vi "ProjectorCameraXY2LinearTransformation.vi"(7 "error in (no error)":errorcluster, 9 "ProjectorXY":cluster{"X":dbl, "Y":dbl}[](graph), 10 "CameraXY":cluster{"X":dbl, "Y":dbl}[](graph)) -> (0 "error out":errorcluster, 3 "Linear Tranformation Description":T1 {"mean error\n(projector pixels)" format="%0.2f"})   [LabVIEW 2019]
uses:
  LinearTransformationDescriptionCluster.ctl
  <vilib>/vision/NI_Vision_Development_Module.lvlib
panel:
  out "CameraXY 3":cluster{"X":dbl, "Y":dbl}[](graph)
  out "ProjectorXY 3":cluster{"X":sgl, "Y":sgl}[](graph)
  out "ProjectorXY 2":cluster{"X":dbl, "Y":dbl}[](graph)
  out "CameraToProjectorCorrectionFactor Y":dbl
  out "CameraToProjectorCorrectionFactor X":dbl
  out "Y axis error":sgl
  out "CameraXY 2":cluster{"X":dbl, "Y":dbl}[](graph)
  out "y axis relative to x":sgl
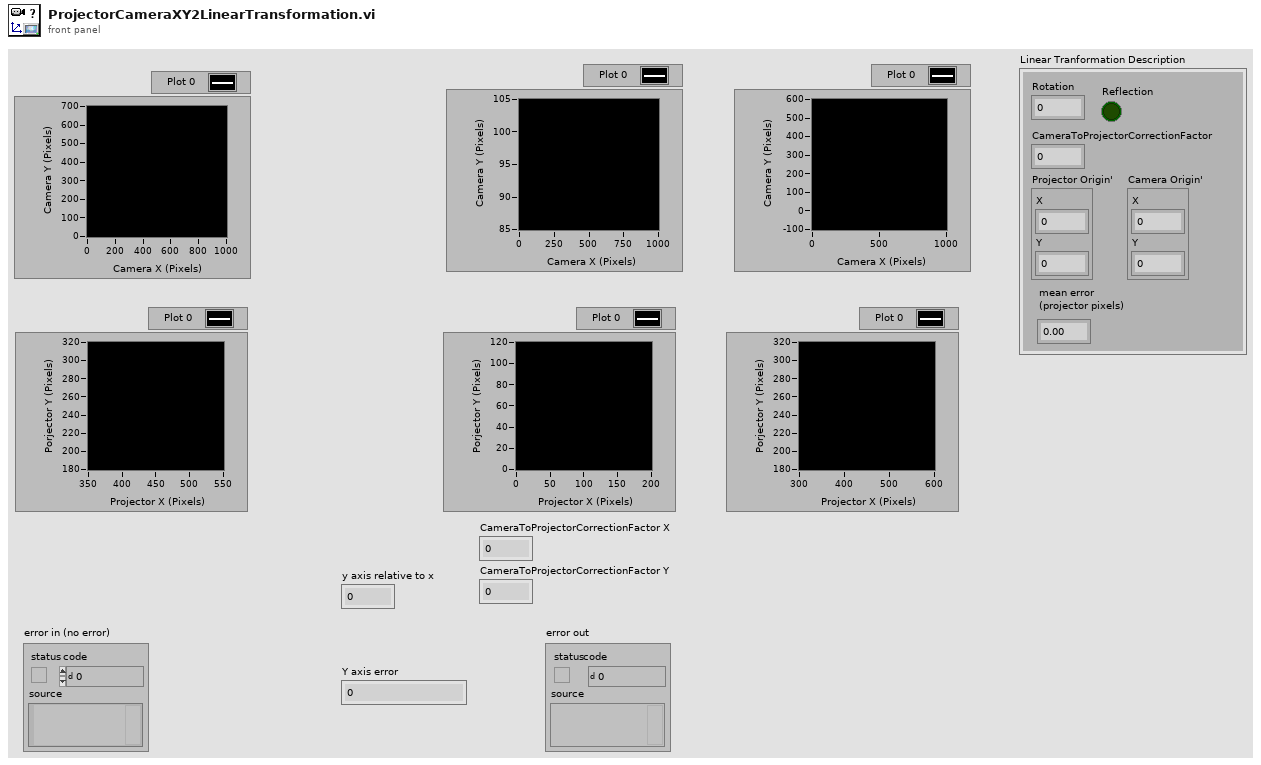
[diagram p1: front panel]
types:
  T1 = typedef "LinearTransformationDescriptionCluster.ctl" = cluster{"Rotation":sgl, "Reflection":bool, "CameraToProjectorCorrectionFactor":dbl, "Projector Origin'":cluster{"X":dbl, "Y":dbl}, "Camera Origin'":cluster{"X":dbl, "Y":dbl}, "mean error\n(projector pixels)":dbl}
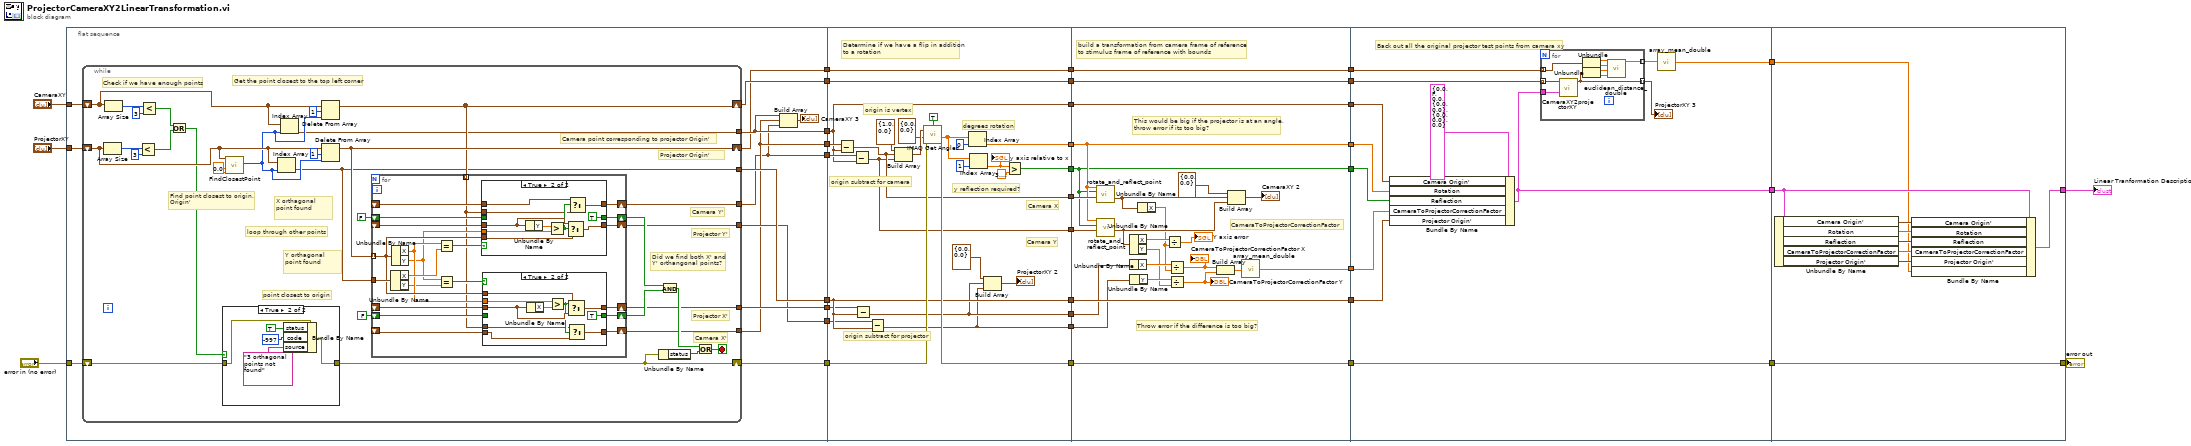
[diagram p0: block diagram]
diagram:
  n1 = flat-sequence {
    tunnel: "CameraXY" -> [w49]
    tunnel: "ProjectorXY" -> [w48]
    tunnel: "error in (no error)" -> [w47]
    tunnel: [w46] -> w32
    tunnel: [w40] -> w31
    tunnel: [w37] -> w30
    tunnel: [w45] -> w29
    tunnel: [w44] -> w28
    tunnel: [w43] -> w27
    tunnel: [w41] -> w25
    tunnel: [w39] -> w10
    tunnel: [w38] -> w7
    tunnel: w32 -> [w146]
    tunnel: w31 -> [w159]
    tunnel: w30 -> [w158]
    tunnel: w29 -> [w141]
    tunnel: w28 -> [w138]
    tunnel: w27 -> [w140]
    tunnel: [w145] -> w26
    tunnel: w25 -> [w142]
    tunnel: [w148] -> w24
    tunnel: [w147] -> w23
    tunnel: [w137] -> w22
    tunnel: [w136] -> w21
    tunnel: [w144] -> w20
    tunnel: [w143] -> w19
    tunnel: [w142] -> w16
    tunnel: [w141] -> w12
    tunnel: w10 -> [w135]
    tunnel: [w135] -> w9
    tunnel: w7 -> [w133]
    tunnel: [w133] -> w5
    tunnel: w26 -> [w184]
    tunnel: w24 -> [w166]
    tunnel: w23 -> [w165]
    tunnel: w22 -> [w163]
    tunnel: w21 -> [w162]
    tunnel: w20 -> [w181]
    tunnel: w19 -> [w180]
    tunnel: [w184] -> w18
    tunnel: [w168] -> w17
    tunnel: w16 -> [w167]
    tunnel: [w167] -> w15
    tunnel: [w166] -> w14
    tunnel: [w165] -> w13
    tunnel: w12 -> [w164]
    tunnel: [w164] -> w11
    tunnel: w9 -> [w161]
    tunnel: [w161] -> w8
    tunnel: [w160] -> w6
    tunnel: w5 -> [w160]
    tunnel: w18 -> [w197]
    tunnel: w17 -> [w189]
    tunnel: w15 -> [w192]
    tunnel: w14 -> [w191]
    tunnel: w13 -> [w190]
    tunnel: w11 -> [w188]
    tunnel: w8 -> [w196]
    tunnel: w6 -> [w194]
    tunnel: [w197] -> w3
    tunnel: [w186] -> w2
    tunnel: [w185] -> w1
    tunnel: [w214] -> w4
    tunnel: [w215] -> w33
    tunnel: w3 -> [w215]
    tunnel: w2 -> [w213]
    tunnel: w1 -> [w207]
    frame #0 {
      n2 = while {
        shift-right: [w76] -> w46
        shift-left: w47 -> [w77]
        shift-right: [w54] -> w39
        shift-left: w49 -> [w79]
        shift-right: [w75] -> w38
        shift-left: w48 -> [w78]
        tunnel: [w56] -> w43
        tunnel: [w55] -> w44
        tunnel: [w53] -> w45
        tunnel: [w52] -> w40
        tunnel: [w51] -> w37
        tunnel: [w50] -> w41
        stop <- w58 stop-if-true
        w74 = 0.0
        # "Find point closest to origin,\nOrigin'"
        # "Did we find both X' and\nY' orthangonal points?"
        # "Camera X'"
        # "Projector X'"
        # "Camera Y'"
        # "Camera point corresponding to projector Origin'"
        # "Projector Y'"
        # "Projector Origin'"
        # "X orthagonal\npoint found"
        # "loop through other points"
        # "point closest to origin"
        # "Y orthagonal\npoint found"
        # "Check if we have enough points"
        # "Get the point closest to the top left corner"
        n3 = Array Size(array=w78) -> (size(s)=w70:i32)
        n4 = Array Size(array=w79) -> (size(s)=w73:i32)
        n5 = Less?(x=w70, y=3) -> (x < y?=w68:bool)
        n6 = Less?(x=w73, y=3) -> (x < y?=w69:bool)
        n7 = Or(x=w69, y=w68) -> (x .or. y?=w60:bool)
        n8 = case shown="True" w60 {
          tunnel: w77 -> [w127 w130]
          tunnel: [w127 w129] -> w76
          frame False {
          }
          frame True {
            n9 = Bundle By Name(cluster=w130, "status"=TRUE, "code"=-997, "source"="3 orthagonal points not found") -> (w129:errorcluster)
          }
        }
        n10 = call "FindClosestPoint.vi"("Y"=w74, "X"=w74, "Points"=w78) -> ("ShortestDistanceIndex"=w65:i32)  [unwired: 7 in, 1 out]
        n11 = Index Array(array=w78, index=w65) -> (element=w53:cluster{"X":dbl, "Y":dbl})
        n12 = Index Array(array=w79, index=w65) -> (element=w50:cluster{"X":dbl, "Y":dbl})
        n13 = Delete From Array(array=w79, length=1, index=w65) -> (array with subset deleted=w54:cluster{"X":dbl, "Y":dbl}[])  [unwired: 1 out]
        n14 = Delete From Array(array=w78, length=1, index=w65) -> (array with subset deleted=w75:cluster{"X":dbl, "Y":dbl}[])  [unwired: 1 out]
        n15 = for {
          tunnel: w75 -> [w88] mode=indexing
          shift-right: [w95] -> w62
          shift-left: FALSE -> [w96]
          shift-right: [w93] -> w56
          shift-left: _ -> [w94]
          tunnel: w53 -> [w100]
          shift-right: [w92] -> w61
          shift-left: FALSE -> [w91]
          shift-right: [w89] -> w55
          shift-left: _ -> [w90]
          tunnel: w54 -> [w80] mode=indexing
          shift-right: [w83] -> w51
          shift-left: _ -> [w84]
          shift-right: [w81] -> w52
          shift-left: _ -> [w82]
          n16 = Unbundle By Name(w100) -> ("X"=w98:dbl, "Y"=w86:dbl)
          n17 = Unbundle By Name(w88) -> ("X"=w87:dbl, "Y"=w85:dbl)
          n18 = Equal?(x=w87, y=w98) -> (x = y?=w99:bool)
          n19 = Equal?(x=w85, y=w86) -> (x = y?=w97:bool)
          n20 = case shown="True" w99 {
            tunnel: w96 -> [w116 _]
            tunnel: [w116 TRUE] -> w95
            tunnel: w94 -> [w115 w122]
            tunnel: [w115 w123] -> w93
            tunnel: w88 -> [_ w121]
            tunnel: w85 -> [_ w124]
            tunnel: w84 -> [w114 w118]
            tunnel: [w114 w120] -> w83
            tunnel: w80 -> [_ w117]
            frame False {
            }
            frame True {
              n21 = Unbundle By Name(w122) -> ("Y"=w125:dbl)
              n22 = Greater?(x=w125, y=w124) -> (0:w119:bool)
              n23 = Select(t=w122, s=w119, f=w121) -> (s? t:f=w123:cluster{"X":dbl, "Y":dbl})
              n24 = Select(t=w118, s=w119, f=w117) -> (s? t:f=w120:cluster{"X":dbl, "Y":dbl})
            }
          }
          n25 = case shown="True" w97 {
            tunnel: [w103 TRUE] -> w92
            tunnel: w91 -> [w103 _]
            tunnel: [w102 w112] -> w89
            tunnel: w90 -> [w102 w110]
            tunnel: w88 -> [_ w108]
            tunnel: w87 -> [_ w109]
            tunnel: w82 -> [w101 w105]
            tunnel: [w101 w107] -> w81
            tunnel: w80 -> [_ w104]
            frame False {
            }
            frame True {
              n26 = Unbundle By Name(w110) -> ("X"=w111:dbl)
              n27 = Greater?(x=w109, y=w111) -> (0:w106:bool)
              n28 = Select(t=w108, s=w106, f=w110) -> (s? t:f=w112:cluster{"X":dbl, "Y":dbl})
              n29 = Select(t=w104, s=w106, f=w105) -> (s? t:f=w107:cluster{"X":dbl, "Y":dbl})
            }
          }
        }
        n30 = Unbundle By Name(w76) -> ("status"=w57:bool)
        n31 = And(x=w62, y=w61) -> (x .and. y?=w59:bool)
        n32 = Or(x=w59, y=w57) -> (x .or. y?=w58:bool)
      }
      n33 = Build Array(w41, w40, w37) -> (→"CameraXY 3":cluster{"X":dbl, "Y":dbl}[])
    }
    frame #1 {
      # "Camera Y"
      # "Camera X"
      # "origin subtract for projector"
      # "Determine if we have a flip in addition\nto a rotation"
      # "y reflection required?"
      # "degrees rotation"
      # "origin is vertex"
      # "origin subtract for camera"
      n34 = Subtract(x=w159, y=w142) -> (x-y=w144:cluster{"X":dbl, "Y":dbl})
      n35 = Subtract(x=w158, y=w142) -> (x-y=w143:cluster{"X":dbl, "Y":dbl})
      n36 = Subtract(x=w138, y=w141) -> (x-y=w137:cluster{"X":dbl, "Y":dbl})
      n37 = Subtract(x=w140, y=w141) -> (x-y=w136:cluster{"X":dbl, "Y":dbl})
      n38 = Build Array(cluster{"X":dbl, "Y":dbl} {"X"=1.0, "Y"=0.0}, w144, w143) -> (w155:cluster{"X":dbl, "Y":dbl}[])
      n39 = call "IMAQ Get Angles"("error in (no error)"=w146, "Vertex"=cluster{"X":dbl, "Y":dbl} {"X"=0.0, "Y"=0.0}, "Points"=w155, "Use Vertex (No)"=TRUE) -> ("error out"=w145:errorcluster, "Angles (rad)"=w151:sgl[])  [unwired: 1 in, 1 out]
      n40 = Index Array(array=w151, index=0) -> (element=w148:sgl)
      n41 = Index Array(array=w151, index=1) -> (element=w150:sgl)
      "y axis relative to x" <- w150
      n42 = Build Array(cluster{"X":dbl, "Y":dbl} {"X"=0.0, "Y"=0.0}, w137, w136) -> (→"ProjectorXY 2":cluster{"X":dbl, "Y":dbl}[])
      n43 = Greater?(x=w150, y=3.141592653589793) -> (0:w147:bool)
    }
    frame #2 {
      # "Throw error if the difference is too big?"
      # "CameraToProjectorCorrectionFactor"
      # "This would be big if the projector is at an angle,\nthrow error if its too big?"
      # "build a transformation from camera frame of reference\nto stimulus frame of reference with bounds"
      n44 = call "rotate_and_reflect_point.vi"("Point"=w181, "reflect about the x axis?"=w165, "rotation angle (radians)"=w166) -> ("transformed point"=w179:cluster{"X":sgl, "Y":sgl})  [unwired: 8 in]
      n45 = call "rotate_and_reflect_point.vi"("Point"=w180, "reflect about the x axis?"=w165, "rotation angle (radians)"=w166) -> ("transformed point"=w178:cluster{"X":sgl, "Y":sgl})  [unwired: 8 in]
      n46 = Unbundle By Name(w178) -> ("X"=w177:sgl, "Y"=w172:sgl)
      n47 = Unbundle By Name(w163) -> ("X"=w175:dbl)
      n48 = Unbundle By Name(w162) -> ("Y"=w173:dbl)
      n49 = Unbundle By Name(w179) -> ("X"=w174:sgl)
      n50 = Divide(x=w177, y=w174) -> (x/y=→"Y axis error":sgl)
      n51 = Divide(x=w175, y=w174) -> (x/y=w170:dbl)
      "CameraToProjectorCorrectionFactor X" <- w170
      n52 = Divide(x=w173, y=w172) -> (x/y=w169:dbl)
      "CameraToProjectorCorrectionFactor Y" <- w169
      n53 = Build Array(w170, w169) -> (w171:dbl[])
      n54 = Build Array(cluster{"X":dbl, "Y":dbl} {"X"=0.0, "Y"=0.0}, w179, w178) -> (→"CameraXY 2":cluster{"X":dbl, "Y":dbl}[])
      n55 = call "array_mean_double.vi"("Input"=w171) -> ("Array Mean"=w168:dbl)
    }
    frame #3 {
      # "Back out all the original projector test points from camera xy"
      n56 = Bundle By Name(cluster=T1 {"Rotation"=0.0, "Reflection"=FALSE, "CameraToProjectorCorrectionFactor"=0.0, "Projector Origin'"={"X"=0.0, "Y"=0.0}, "Camera Origin'"={"X"=0.0, "Y"=0.0}, "mean error\n(projector pixels)"=0.0} ("Linear Transformation Description Template"), "Camera Origin'"=w192, "Rotation"=w191, "Reflection"=w190, "CameraToProjectorCorrectionFactor"=w189, "Projector Origin'"=w188) -> (w186:T1)
      n57 = for {
        tunnel: w196 -> [w206] mode=indexing
        tunnel: [w204] -> w195 mode=indexing
        tunnel: w194 -> [w205] mode=indexing
        tunnel: [w199] -> w193 mode=indexing
        tunnel: w186 -> [w198]
        n58 = call "CameraXY2projectorXY.vi"("Linear Transformation Description"=w198, "Camera Point"=w206) -> ("Projector Point"=w204:cluster{"X":sgl, "Y":sgl})  [unwired: 9 in]
        n59 = Unbundle(w205) -> ("X"=w203:dbl, "Y"=w202:dbl)
        n60 = Unbundle(w204) -> ("X"=w201:sgl, "Y"=w200:sgl)
        n61 = call "euclidean_distance_double.vi"("Point 2 Y"=w200, "Point 2 X"=w201, "Point 1 Y"=w202, "Point 1 X"=w203) -> ("Distance"=w199:dbl)  [unwired: 7 in]
      }
      "ProjectorXY 3" <- w195
      n62 = call "array_mean_double.vi"("Input"=w193) -> ("Array Mean"=w185:dbl)
    }
    frame #4 {
      n63 = Unbundle By Name(w213) -> ("Camera Origin'"=w212:cluster{"X":dbl, "Y":dbl}, "Rotation"=w211:sgl, "Reflection"=w210:bool, "CameraToProjectorCorrectionFactor"=w209:dbl, "Projector Origin'"=w208:cluster{"X":dbl, "Y":dbl})
      n64 = Bundle By Name(cluster=w213, "Camera Origin'"=w212, "Rotation"=w211, "Reflection"=w210, "CameraToProjectorCorrectionFactor"=w209, "Projector Origin'"=w208, "mean error\n(projector pixels)"=w207) -> (w214:T1)
    }
  }
  "error out" <- w33
  "Linear Tranformation Description" <- w4
